vi "BumpIntakeLogic.vi"(1 "Command":bool) -> (0 "Auto_Bump_Intake":bool)   [LabVIEW 2019]
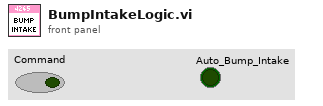
[diagram p1: front panel]
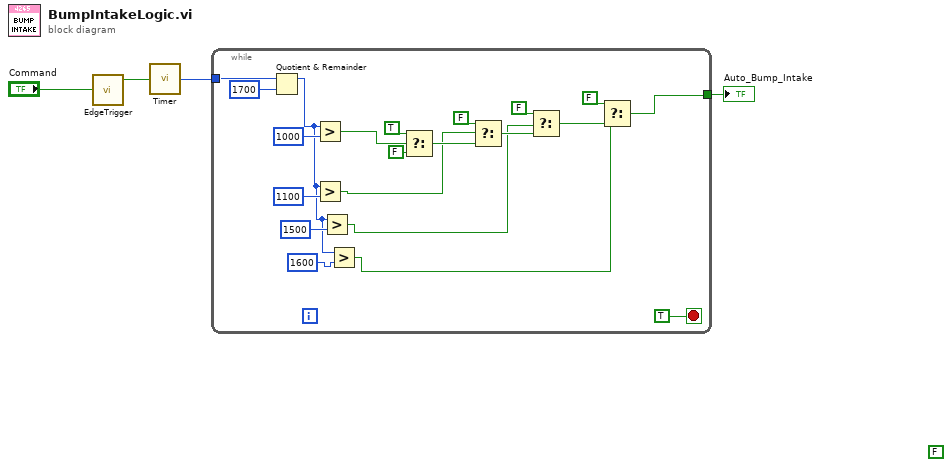
[diagram p0: block diagram]
diagram:
  (unwired) FALSE
  n1 = call "EdgeTrigger.vi"("Input Signal"="Command") -> ("Rising Edge Trigger"=w3:bool)  [unwired: 2 out]
  n2 = call "Timer.vi"("Reset Timer"=w3) -> ("Time (ms)"=w2:u32)
  n3 = while {
    tunnel: w2 -> [w14]
    tunnel: [w17] -> w1
    stop <- TRUE stop-if-true
    n4 = Quotient & Remainder(x=w14, y=u32 1700) -> (x-y*floor(x/y)=w8:u32)  [unwired: 1 out]
    n5 = Greater?(x=w8, y=u32 1000) -> (0:w12:bool)
    n6 = Greater?(x=w8, y=u32 1100) -> (0:w7:bool)
    n7 = Greater?(x=w8, y=u32 1500) -> (0:w6:bool)
    n8 = Greater?(x=w8, y=u32 1600) -> (0:w5:bool)
    n9 = Select(t=TRUE, s=w12, f=FALSE) -> (s? t:f=w21:bool)
    n10 = Select(t=FALSE, s=w7, f=w21) -> (s? t:f=w20:bool)
    n11 = Select(t=FALSE, s=w6, f=w20) -> (s? t:f=w18:bool)
    n12 = Select(t=FALSE, s=w5, f=w18) -> (s? t:f=w17:bool)
  }
  "Auto_Bump_Intake" <- w1
